vi "Vision Testing.vi"(7 "error in":errorcluster) -> (20 "Image Out":T3(plugin-control), 27 "error out":errorcluster)   [LabVIEW 2015]
doc: "Creates, and edits acquisitions using the NI Vision Acquisition Express VI.\n\nThe NI Vision Acquisition Wizard is launched by placing the Express VI on the block diagram. Select an acquisition source and configure an acquisition using NI-IMAQ, NI-IMAQdx, or simulate an acquisition by reading an AVI or image files from a folder. After an acquisition is configured, select controls and indicators to be able to programmatically set in LabVIEW. Double-click the Vision Acquisition Express VI to edit the acquisition.\n\nNote: Any images created by the Express VI need to be disposed after use. Use the IMAQ Dispose.vi to cleanup the images output by the Express VI when they are no longer needed."
uses:
  <vilib>/vision/Image Controls.llb/IMAQ Image.ctl
  <vilib>/vision/driver/IMAQdx.llb/IMAQdx Attribute Type.ctl
panel:
  in  "Interface Name":string="cam1"
  out "Attribute Information Array":T2(array[cluster])
  out "concatenated string":string
  in  "Attributes":string="[NIIMAQ_HEADER]\nType = 2\nVersion = 8\n\n[CAMERA_DATA]\nAcquisitionAttributes::Bayer::GainB = \"1\"\nAcquisitionAttributes::Bayer::GainG = \"1\"\nAcquisitionAttributes::Bayer::GainR = \"1\"\nAcquisitionAttributes::Bayer::Pattern = \"Use hardware value\"\nAcquisitionAttributes::BitsPerPixel = \"Use hardware value\"\nAcquisitionAttributes::IgnoreFirstFrame = \"false\"\nAcquisitionAttributes::OverwriteMode = \"Get Newest\"\nAcquisitionAttributes::PixelSignedness = \"Signed\"\nAcquisitionAttributes::ReceiveTimestampMode = \"None\"\nAcquisitionAttributes::ShiftPixelBits = \"false\"\nAcquisitionAttributes::SwapPixelBytes = \"false\"\nAcquisitionAttributes::Timeout = \"5000\"\nAcquisitionAttributes::VerticalMirror = \"false\"\nAcquisitionAttributes::VideoMode = \"1280x1024 RGB24 5.00fps\"\nCameraAttributes::BacklightCompensation::Mode = \"Manual\"\nCameraAttributes::BacklightCompensation::Value = \"true\"\nCameraAttributes::Brightness::Mode = \"Manual\"\nCameraAttributes::Brightness::Value = \"144\"\nCameraAttributes::Contrast::Mode = \"Manual\"\nCameraAttributes::Contrast::Value = \"0.27000000000000002\"\nCameraAttributes::Exposure::Mode = \"Auto\"\nCameraAttributes::Gain::Mode = \"Manual\"\nCameraAttributes::Gain::Value = \"10\"\nCameraAttributes::Saturation::Mode = \"Manual\"\nCameraAttributes::Saturation::Value = \"28\"\nCameraAttributes::Sharpness::Mode = \"Manual\"\nCameraAttributes::Sharpness::Value = \"180\"\nCameraAttributes::WhiteBalance::Mode = \"Manual\"\nCameraAttributes::WhiteBalance::Value = \"5511\"\n"
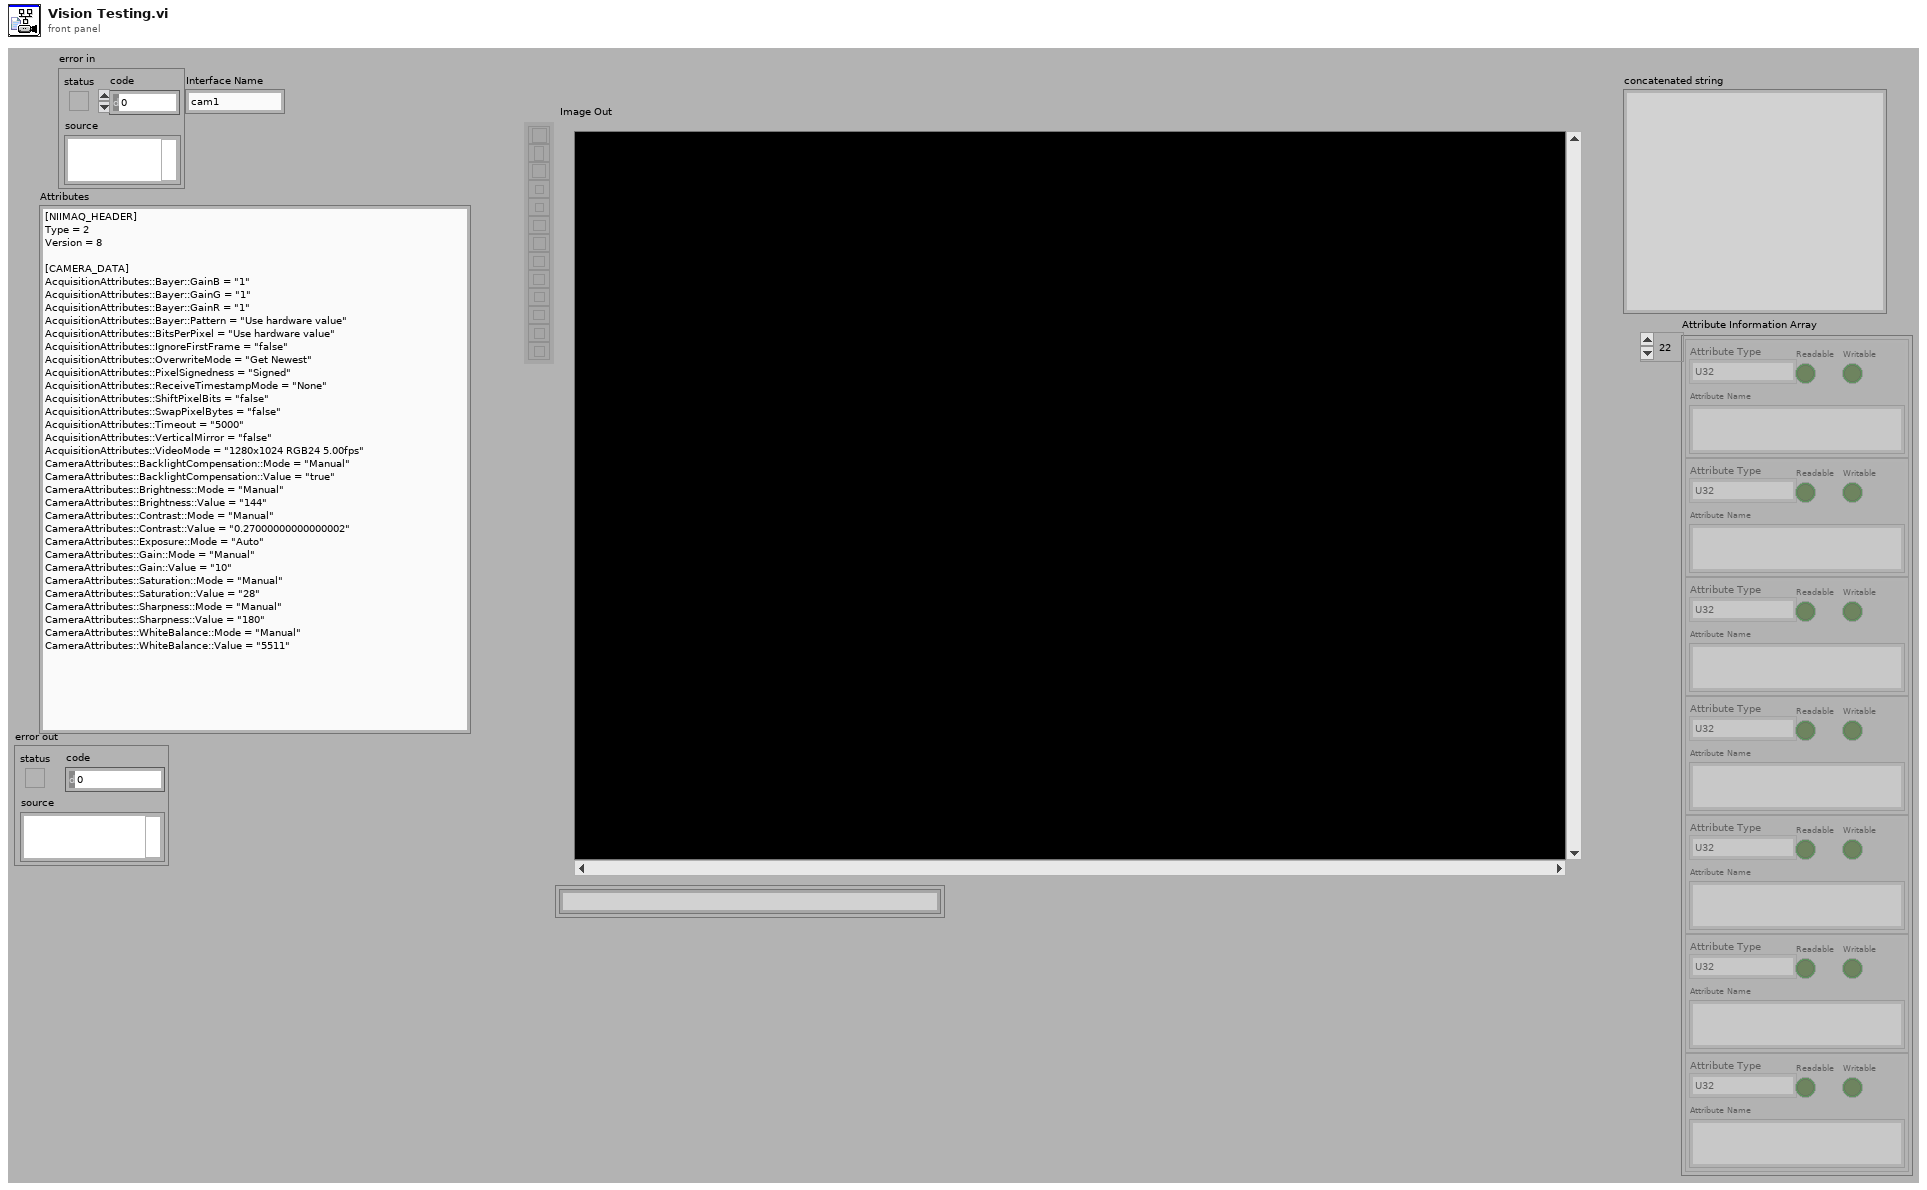
[diagram p1: front panel]
types:
  T1 = typedef "NI_Vision_Acquisition_Software.lvlib/IMAQdx Attribute Type.ctl" = enum32{"U32", "I64", "DBL", "String", "Enum", "Bool", "Command"}
  T2 = cluster{"Attribute Type":T1, "Readable":bool, "Writable":bool, "Attribute Name":string}[]
  T3 = typedef "IMAQ Image.ctl" = refnum<image>
  T4 = typedef "IMAQdx.ctl" = refnum<k21>
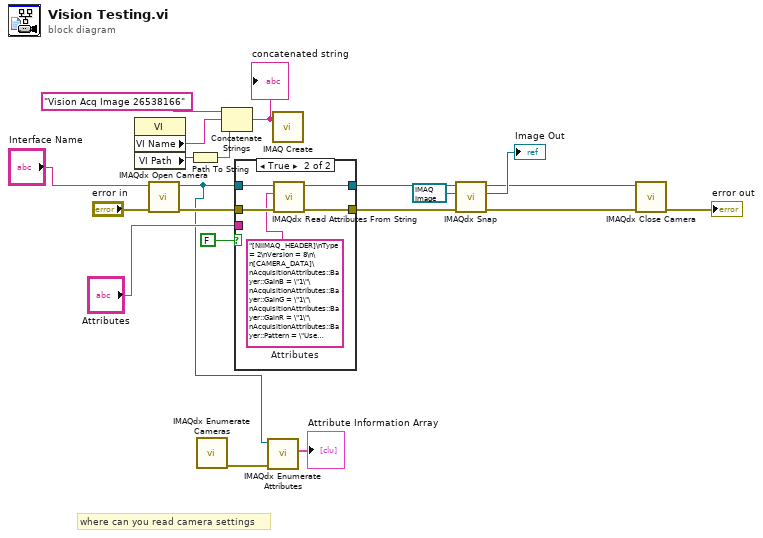
[diagram p0: block diagram]
diagram:
  # "where can you read camera settings"
  n1 = property class="VI"() -> ("VI Name"=w18:string, "VI Path"=w19:path)  [unwired: 2 in, 2 out]
  n2 = call <vilib>:"IMAQdx Open Camera.vi"("error in"="error in", "Session In"="Interface Name") -> ("error out"=w14:errorcluster, "Session Out"=w2:T4)  [unwired: 1 in, 7 out]
  n3 = Path To String(path=w19) -> (string=w17:string)
  n4 = call <vilib>:"IMAQdx Enumerate Cameras.vi"() -> ("error out"=w5:errorcluster)  [unwired: 10 in, 1 out]
  n5 = Concatenate Strings("Vision Acq Image 26538166" ("Image Name"), w18, w17) -> (w15:string)
  "concatenated string" <- w15
  n6 = case shown="True" FALSE ("Init Attributes") {
    tunnel: w2 -> [w22 w27]
    tunnel: w14 -> [w21 w26]
    tunnel: [w22 w25] -> w9
    tunnel: [w21 w24] -> w13
    tunnel: "Attributes" -> [_ _]
    frame False {
    }
    frame True {
      w23 = "[NIIMAQ_HEADER]\nType = 2\nVersion = 8\n\n[CAMERA_DATA]\nAcquisitionAttributes::Bayer::GainB = \"1\"\nAcquisitionAttributes::Bayer::GainG = \"1\"\nAcquisitionAttributes::Bayer::GainR = \"1\"\nAcquisitionAttributes::Bayer::Pattern = \"Use hardware value\"\nAcquisitionAttributes::BitsPerPixel = \"Use hardware value\"\nAcquisitionAttributes::IgnoreFirstFrame = \"false\"\nAcquisitionAttributes::OverwriteMode = \"Get Newest\"\nAcquisitionAttributes::PixelSignedness = \"Signed\"\nAcquisitionAttributes::ReceiveTimestampMode = \"None\"\nAcquisitionAttributes::ShiftPixelBits = \"false\"\nAcquisitionAttributes::SwapPixelBytes = \"false\"\nAcquisitionAttributes::Timeout = \"5000\"\nAcquisitionAttributes::VerticalMirror = \"false\"\nAcquisitionAttributes::VideoMode = \"1280x1024 RGB24 5.00fps\"\nCameraAttributes::BacklightCompensation::Mode = \"Manual\"\nCameraAttributes::BacklightCompensation::Value = \"true\"\nCameraAttributes::Brightness::Mode = \"Manual\"\nCameraAttributes::Brightness::Value = \"144\"\nCameraAttributes::Contrast::Mode = \"Manual\"\nCameraAttributes::Contrast::Value = \"0.27000000000000002\"\nCameraAttributes::Exposure::Mode = \"Auto\"\nCameraAttributes::Gain::Mode = \"Manual\"\nCameraAttributes::Gain::Value = \"10\"\nCameraAttributes::Saturation::Mode = \"Manual\"\nCameraAttributes::Saturation::Value = \"28\"\nCameraAttributes::Sharpness::Mode = \"Manual\"\nCameraAttributes::Sharpness::Value = \"180\"\nCameraAttributes::WhiteBalance::Mode = \"Manual\"\nCameraAttributes::WhiteBalance::Value = \"5511\"\n"  # Attributes
      n7 = call <vilib>:"IMAQdx Read Attributes From String.vi"("error in"=w26, "Attributes String In"=w23, "Session In"=w27) -> ("error out"=w24:errorcluster, "Session Out"=w25:T4)  [unwired: 7 out]
    }
  }
  n8 = call <vilib>:"IMAQdx Enumerate Attributes.vi"("error in"=w5, "Session In"=w2) -> ("Attribute Information Array"=→"Attribute Information Array":T2)  [unwired: 7 in, 2 out]
  n9 = call "IMAQ Create"("Image Name"=w15) -> ()  [unwired: 3 in, 3 out]
  n10 = call <vilib>:"IMAQdx Snap.vi"("error in"=w13, "Image In"=T3 refnum, "Session In"=w9) -> ("error out"=w11:errorcluster, "Image Out"=→"Image Out":T3, "Session Out"=w7:T4)  [unwired: 6 out]
  n11 = call <vilib>:"IMAQdx Close Camera.vi"("error in"=w11, "Session In"=w7) -> ("error out"=→"error out":errorcluster)  [unwired: 9 out]
